vi "Training.vi"   [LabVIEW 2013]
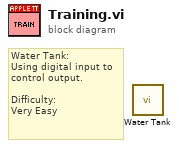
[diagram p0: block diagram]
diagram:
  # "Water Tank:\nUsing digital input to\ncontrol output.\n\nDifficulty:\nVery Easy"
  n1 = call "Water Tank.vi"() -> ()  [unwired: 1 out]
